vi "Collect_Ref_Signal.vi"(4 "ref device name":tag="Dev2", 6 "error in":errorcluster, 8 "Reference Sample Rate (Hz)":dbl=2000.0, 9 "Inner Loop Run Time":dbl, 10 "Working Directory":string, 11 "Inner Loop Ended?":bool) -> (0 "error out":errorcluster)   [LabVIEW 2012]
uses:
  <vilib>/Utility/file.llb/Write To Spreadsheet File (DBL).vi
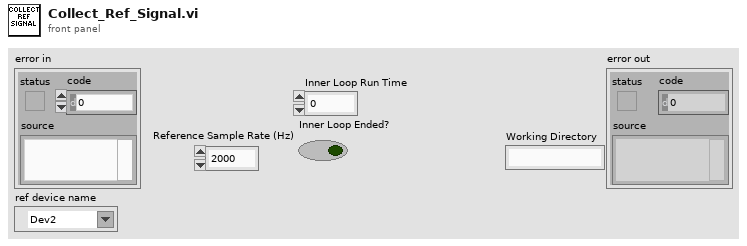
[diagram p1: front panel]
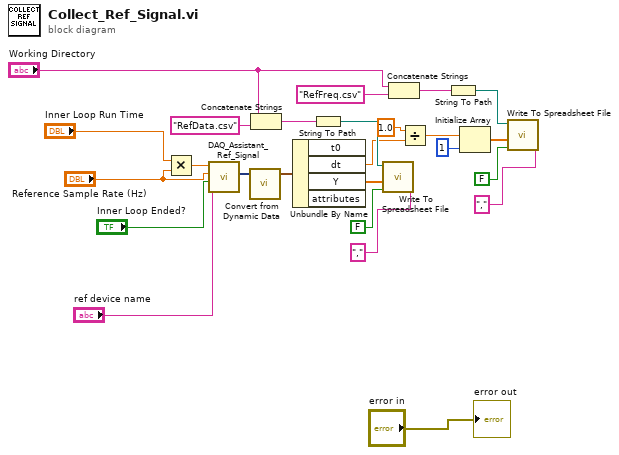
[diagram p0: block diagram]
diagram:
  n1 = Multiply(x="Inner Loop Run Time", y="Reference Sample Rate (Hz)") -> (x*y=w10:dbl)
  n2 = call "DAQ_Assistant_Ref_Signal.vi"("device name"="ref device name", "stop (F)"="Inner Loop Ended?", "rate"="Reference Sample Rate (Hz)", "number of samples"=w10) -> ("data 2"=w25:dynamicdata)  [unwired: 7 in]
  n3 = call "Convert from Dynamic Data"("Dynamic Data Type"=w25) -> ("Waveform"=w24:waveform(dbl))  [unwired: 3 in]
  n4 = Concatenate Strings("Working Directory", "RefData.csv") -> (w8:string)
  n5 = Unbundle By Name(w24) -> ("dt"=w19:dbl, "Y"=w21:dbl[])  [unwired: 2 out]
  n6 = String To Path(string=w8) -> (path=w20:path)
  n7 = call-poly <vilib>:"Write To Spreadsheet File.vi"("delimiter (\\t)"=",", "append to file? (new file:F)"=FALSE, "1D data"=w21, "file path (dialog if empty)"=w20) -> ()  [unwired: 4 in, 1 out]
  n8 = Concatenate Strings("Working Directory", "RefFreq.csv") -> (w6:string)
  n9 = Divide(x=1.0, y=w19) -> (x/y=w14:dbl)
  n10 = String To Path(string=w6) -> (path=w15:path)
  n11 = Initialize Array(w14, 1 ("dimension size")) -> (w12:dbl[])
  n12 = call-poly <vilib>:"Write To Spreadsheet File.vi"("delimiter (\\t)"=",", "append to file? (new file:F)"=FALSE, "1D data"=w12, "file path (dialog if empty)"=w15) -> ()  [unwired: 4 in, 1 out]
  "error out" <- "error in"
